vi "rs3 set ROI 3.vi"(4 "max_y":i32, 5 "max_x":i32, 6 "min_y":i32, 7 "min_x":i32, 8 "error in (no error)":errorcluster, 11 "Sensor in":u64) -> (0 "error out":errorcluster, 1 "error":u64, 3 "Sensor out":u64)   [LabVIEW 2017, in "libRealSense3.lvlib"]
doc: "Sets the value of a specific device option\n \nInput:\noption the option whose value to set\nvalue the desired value to set\n \nOutput:\nerror if non-null, receives any error that occurs during this call, otherwise, errors are ignored"
uses:
  libRealSense3.lvlib
  realsense2.dll
panel:
  # "RS2 Set ROI for Autoexposure"
  # "(C) 2016 Intel Corp.,  AGJ"
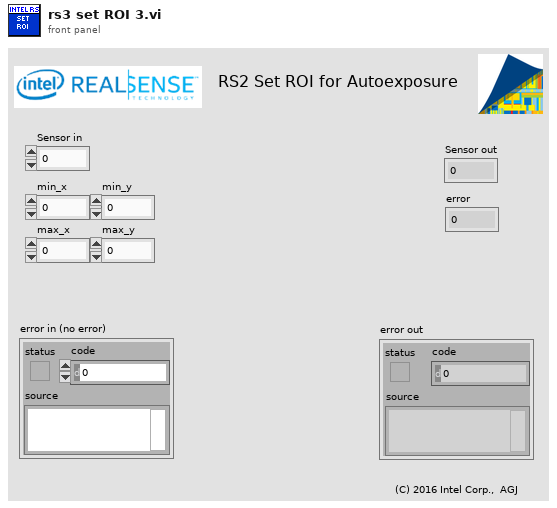
[diagram p1: front panel]
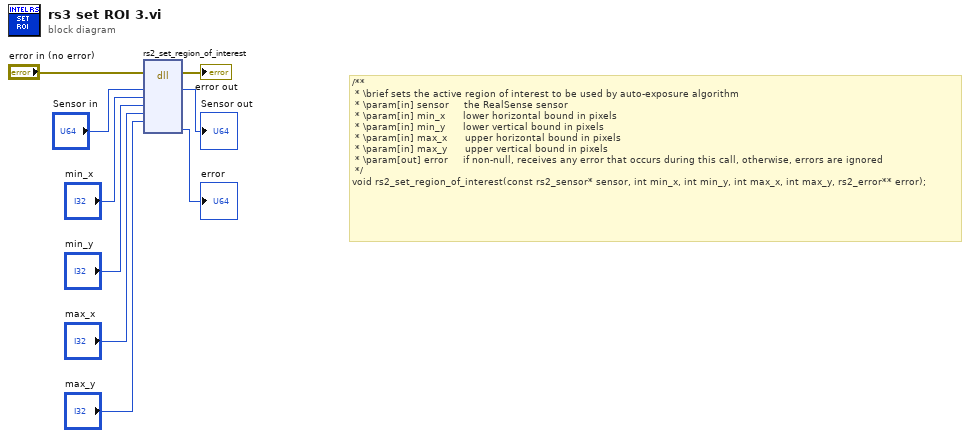
[diagram p0: block diagram]
diagram:
  # "/**\n * \\brief sets the active region of interest to be used by auto-exposure algorithm\n * \\param[in] sensor     the RealSense sensor\n * \\param[in] min_x      lower horizontal bound in pixels\n * \\param[in] min_y      lower vertical bound in pixels\n * \\param[in] max_x      upper horizontal bound in pixels\n * \\param[in] max_y      upper vertical bound in pixels\n * \\param[out] error     if non-null, receives any error that occurs during this call, otherwise, errors are ignored\n */\nvoid rs2_set_region_of_interest(const rs2_sensor* sensor, int min_x, int min_y, int max_x, int max_y, rs2_error** error);"
  n1 = dll-call lib="C:/Users/agrunnet/Documents/libRealSense6/realsense2.dll" fn="rs2_set_region_of_interest"(error in="error in (no error)", "Sensor"="Sensor in", "min_x"="min_x", "min_y"="min_y", "max_x"="max_x", "max_y"="max_y") -> (error out=→"error out":errorcluster, "Sensor"=→"Sensor out":u64, "error"=→"error":u64)  [unwired: 8 in, 1 out]
